vi "DWarns.vi"(11 "End Caching (false)":bool) -> (3 "DWarn Buffer":string)   [LabVIEW 2022 SP3]
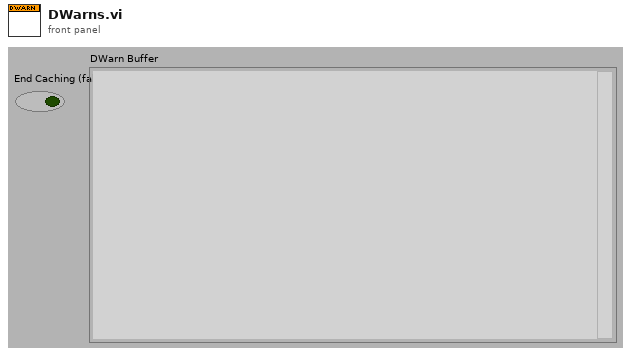
[diagram p1: front panel]
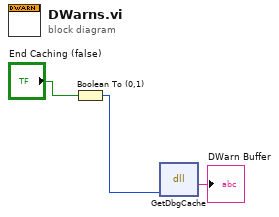
[diagram p0: block diagram]
diagram:
  n1 = Boolean To (0,1)(Boolean="End Caching (false)") -> (0, 1=w2:i16)
  n2 = dll-call lib="LabVIEW" fn="GetDbgCache"("endCaching"=w2) -> ("DWarn Buffer"=→"DWarn Buffer":string)  [unwired: 4 in, 2 out]
